vi "test_ccd_centerWavelength.vi"(8 "error in":errorcluster, 11 "CCD in":refnum<class "CCD.lvclass">) -> (0 "error out":errorcluster, 3 "CCD out":refnum<class "CCD.lvclass">)   [LabVIEW 2023, in "horiba.test.lvlib"]
uses:
  horiba.test.lvlib
  Classes/CCD/CCD.lvclass
  <vilib>/addons/_JKI Toolkits/Caraya/classes/Test/Test.lvclass
  <vilib>/addons/_JKI Toolkits/Caraya/classes/Assert/Assert.lvclass
  <userlib>/_OpenG.lib/lvdata/lvdata.llb/openg_variant.lvlib
panel:
  # "Connector Pane"
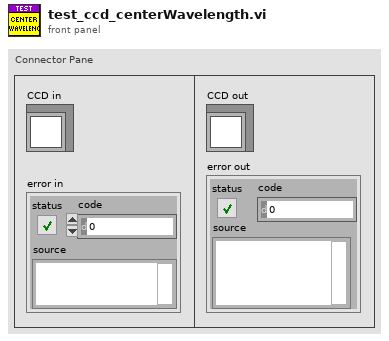
[diagram p1: front panel]
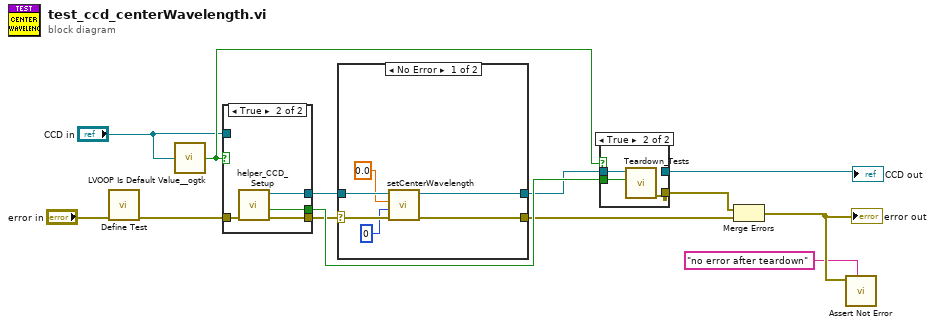
[diagram p0: block diagram]
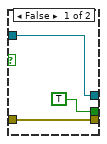
[diagram p2: hidden frame]
diagram:
  n1 = call <vilib>:"Define Test.vi"("error in (no error)"="error in") -> ("error out"=w8:errorcluster)  [unwired: 9 in, 1 out]
  n2 = call <userlib>:"LVOOP Is Default Value__ogtk.vi"("Object"="CCD in") -> ("Is Default Value?"=w9:bool)
  n3 = case shown="True" w9 {
    tunnel: w8 -> [w15 w20]
    tunnel: [w15 w19] -> w4
    tunnel: [w16 w18] -> w6
    tunnel: [TRUE ("Module Was Already Running?") w17] -> w10
    tunnel: "CCD in" -> [w16 _]
    frame False {
    }
    frame True {
      n4 = call "helper_CCD_Setup.vi"("error in"=w20) -> ("error out"=w19:errorcluster, "Module Was Already Running?"=w17:bool, "CCD out"=w18:refnum<class "CCD.lvclass">)  [unwired: 7 in, 1 out]
    }
  }
  n5 = case shown="No Error" w4 {
    selector: w4 -> [w26 w27]
    tunnel: [w25 w28] -> w5
    tunnel: w6 -> [w23 w28]
    tunnel: [w24 w27] -> w3
    frame No Error {
      n6 = call "setCenterWavelength.vi"("error in (no error)"=w26, "monoIndex"=0, "wavelength"=0.0, "CCD in"=w23) -> ("error out"=w24:errorcluster, "CCD out"=w25:refnum<class "CCD.lvclass">)  [unwired: 4 in, 2 out]
    }
    frame Error {
    }
  }
  n7 = case shown="True" w9 {
    tunnel: w5 -> [w29 w32]
    tunnel: [_ w31] -> w7
    tunnel: w10 -> [_ w30]
    tunnel: [w29 _] -> w1
    frame False {
    }
    frame True {
      n8 = call "Teardown_Tests.vi"("Module Was Already Running?"=w30, "horiba.lvlib:GenericDevice"=w32) -> ("error out"=w31:errorcluster)  [unwired: 8 in, 1 out]
    }
  }
  "CCD out" <- w1
  n9 = Merge Errors(w7, w3) -> (w12:errorcluster)
  "error out" <- w12
  n10 = call <vilib>:"Assert Not Error.vi"("Label"="no error after teardown", "Not Error?"=w12) -> ()  [unwired: 8 in, 2 out]
